vi "SiosIfmResetDevice.vi"(0 "Device Number":i32) -> ()   [LabVIEW 2009]
uses:
  siosifm.dll
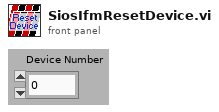
[diagram p1: front panel]
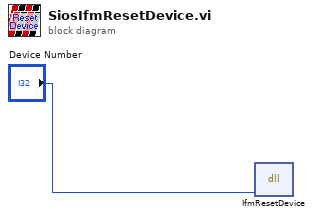
[diagram p0: block diagram]
diagram:
  n1 = dll-call lib="C:/WORK/Artem/RE-10/SIOS_IfmDLL/siosifm.dll" fn="IfmResetDevice"("devNumber"="Device Number") -> ()  [unwired: 5 in, 2 out]
